vi "lua_resume.vi"(7 "from_p":u64, 8 "error in (no error)":errorcluster, 10 "nargs":i32, 11 "lua_state_p":u64) -> (0 "error out":errorcluster, 1 "done?":bool, 3 "lua_state_p out":u64, 5 "nresults":i32)   [LabVIEW 2020, in "lua.dll.lvlib"]
uses:
  lua.dll.lvlib
  lua_thread_status.ctl
  lua_settop.vi
  lua54.dll
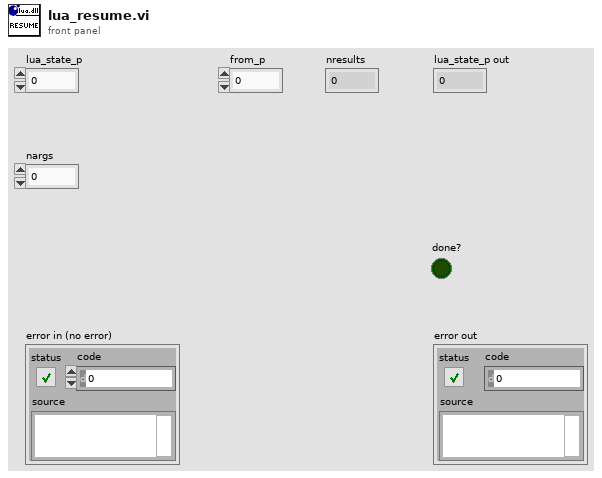
[diagram p1: front panel]
types:
  T1 = typedef "lua.dll.lvlib/lua_thread_status.ctl" = enum8{"LUA_OK", "LUA_YIELD", "LUA_ERRRUN", "LUA_ERRSYNTAX", "LUA_ERRMEM", "LUA_ERRERR"}
  T2 = typedef "lua.dll.lvlib/lua_types.ctl" = i32
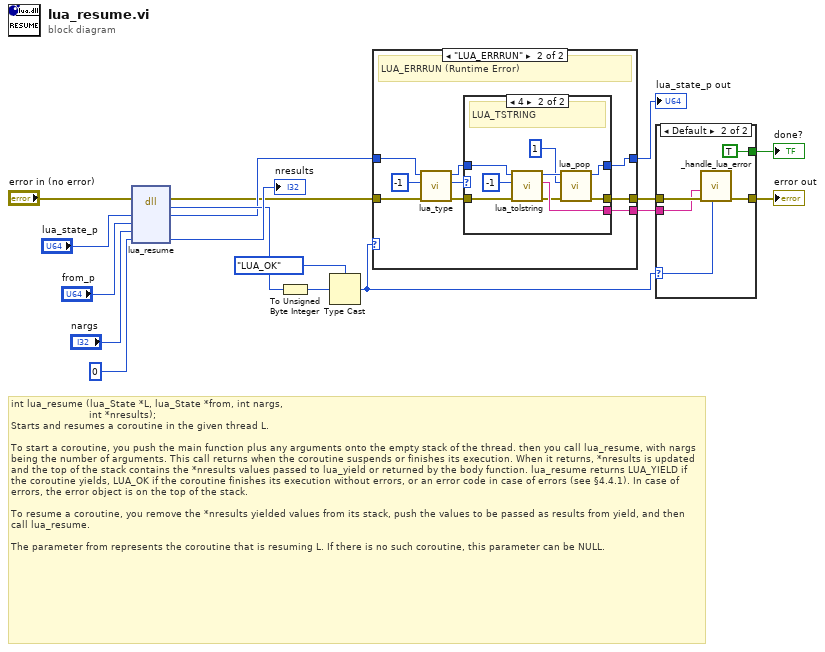
[diagram p0: block diagram]
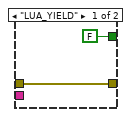
[diagram p4: hidden frame]
diagram:
  # "int lua_resume (lua_State *L, lua_State *from, int nargs,\n                          int *nresults);\nStarts and resumes a coroutine in the given thread L.\n\nTo start a coroutine, you push the main function plus any arguments onto the empty stack of the thread. then you call lua_resume, with nargs being the number of arguments. This call returns when the coroutine suspends or finishes its execution. When it returns, *nresults is updated and the top of the stack contains the *nresults values passed to lua_yield or returned by the body function. lua_resume returns LUA_YIELD if the coroutine yields, LUA_OK if the coroutine finishes its execution without errors, or an error code in case of errors (see §4.4.1). In case of errors, the error object is on the top of the stack.\n\nTo resume a coroutine, you remove the *nresults yielded values from its stack, push the values to be passed as results from yield, and then call lua_resume.\n\nThe parameter from represents the coroutine that is resuming L. If there is no such coroutine, this parameter can be NULL."
  n1 = dll-call lib="C:/Users/Nicholas Folse/Documents/workspace/github-tauterra.llc/Lua for LabVIEW/lib/lua.dll/lua54**.*" fn="lua_resume"(error in="error in (no error)", "lua_state_p"="lua_state_p", "from_p"="from_p", "nargs"="nargs", "nresults"=0) -> (error out=w1:errorcluster, "err_code"=w8:i32, "lua_state_p"=w5:u64, "nresults"=→"nresults":i32)  [unwired: 4 in, 1 out]
  n2 = To Unsigned Byte Integer(number=w8) -> (unsigned 8bit integer=w10:u8)
  n3 = Type Cast(type=lua_thread_status."LUA_OK" ("lua status"), x=w10) -> (*(type *) &x=w6:T1)
  n4 = case shown="\"LUA_ERRRUN\"" w6 {
    tunnel: w5 -> [w19 w25]
    tunnel: [w19 w27] -> w4
    tunnel: [_ w28] -> w3
    tunnel: w1 -> [w18 w24]
    tunnel: [w18 w26] -> w2
    frame Default {
    }
    frame "LUA_ERRRUN" {
      # "LUA_ERRRUN (Runtime Error)"
      n5 = call "lua_type.vi"("error in (no error)"=w24, "index"=-1, "lua_state_p"=w25) -> ("error out"=w21:errorcluster, "lua type"=w20:T2, "lua_state_p out"=w22:u64)  [unwired: 6 in]
      n6 = case shown="4" w20 {
        tunnel: [_ w38] -> w28
        tunnel: [w30 w36] -> w27
        tunnel: [w29 w34] -> w26
        tunnel: w22 -> [w30 w32]
        tunnel: w21 -> [w29 w31]
        frame Default {
        }
        frame 4 {
          # "LUA_TSTRING"
          n7 = call "lua_tolstring.vi"("error in (no error)"=w31, "index"=-1, "lua_state_p"=w32) -> ("error out"=w35:errorcluster, "string"=w38:string, "lua_state_p out"=w37:u64)  [unwired: 6 in]
          n8 = call "lua_pop.vi"("error in (no error)"=w35, "n"=1, "lua_state_p"=w37) -> ("error out"=w34:errorcluster, "lua_state_p out"=w36:u64)  [unwired: 7 in]
        }
      }
    }
  }
  "lua_state_p out" <- w4
  n9 = case shown="Default" w6 {
    selector: w6 -> [_ w44]
    tunnel: [w41 w46] -> w14
    tunnel: w2 -> [w41 w45]
    tunnel: [FALSE TRUE] -> w7
    tunnel: w3 -> [_ w42]
    frame "LUA_YIELD" {
    }
    frame Default {
      n10 = call "_handle_lua_error.vi"("lua status"=w44, "error in (no error)"=w45, "error string"=w42) -> ("error out"=w46:errorcluster)  [unwired: 8 in]
    }
  }
  "error out" <- w14
  "done?" <- w7
